vi "Initialize.vi"(7 "ProjectItem":refnum<class "ProjectItem.lvclass">, 8 "error in (no error)":errorcluster, 10 "New Name":string="NewName", 11 "Pattern":string="[Rename]") -> (0 "error out":errorcluster, 3 "ProjectItem out":refnum<class "ProjectItem.lvclass">)   [LabVIEW 2019, in "ProjectItem.lvclass"]
uses:
  ProjectItem.lvclass
  ProjectItem.lvclass/ProjectItem.ctl
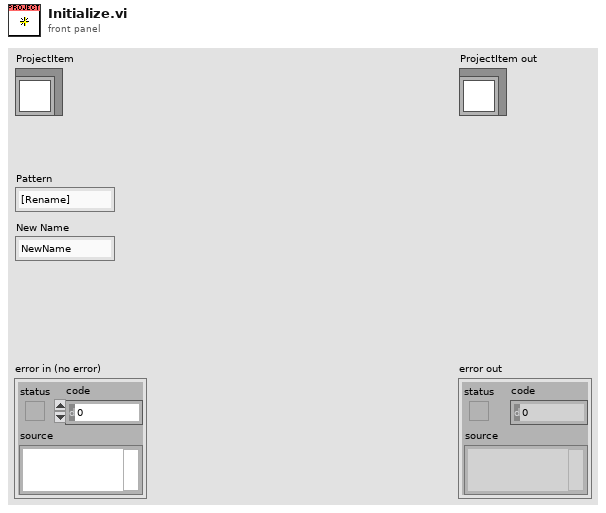
[diagram p1: front panel]
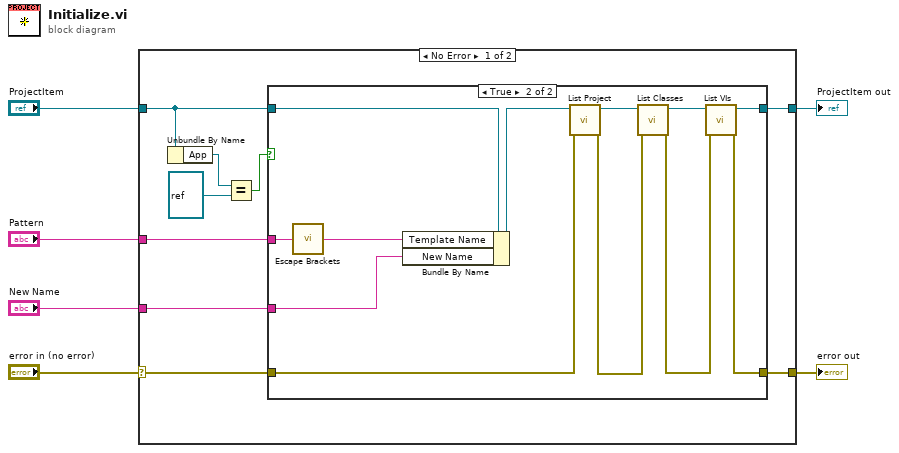
[diagram p0: block diagram]
diagram:
  n1 = case shown="No Error" "error in (no error)" {
    selector: "error in (no error)" -> [w15 w31]
    tunnel: [w13 w31] -> w5
    tunnel: [w14 w30] -> w3
    tunnel: "ProjectItem" -> [w10 w30]
    tunnel: "Pattern" -> [w12 _]
    tunnel: "New Name" -> [w11 _]
    frame No Error {
      n2 = Unbundle By Name(w10) -> ("App"=w9:refnum<vi>)
      n3 = Equal?(x=w9, y=refnum<vi> refnum ("App")) -> (x = y?=w8:bool)
      n4 = case shown="True" w8 {
        tunnel: w15 -> [w16 w21]
        tunnel: [w17 w26] -> w14
        tunnel: [w16 w24] -> w13
        tunnel: w12 -> [_ w29]
        tunnel: w11 -> [_ w18]
        tunnel: w10 -> [w17 w20]
        frame False {
        }
        frame True {
          n5 = call "Escape Brackets.vi"("Pattern"=w29) -> ("result string"=w22:string)
          n6 = Bundle By Name(cluster=w20, "Template Name"=w22, "New Name"=w18) -> (w19:refnum<class "ProjectItem.lvclass">)
          n7 = call "List Project.vi"("error in (no error)"=w21, "Rename in"=w19) -> ("error out"=w23:errorcluster, "Rename out"=w28:refnum<class "ProjectItem.lvclass">)  [unwired: 8 in]
          n8 = call "List Classes.vi"("error in (no error)"=w23, "Rename in"=w28) -> ("error out"=w25:errorcluster, "Rename out"=w27:refnum<class "ProjectItem.lvclass">)  [unwired: 8 in]
          n9 = call "List VIs.vi"("error in (no error)"=w25, "Rename in"=w27) -> ("error out"=w24:errorcluster, "Rename out"=w26:refnum<class "ProjectItem.lvclass">)  [unwired: 8 in]
        }
      }
    }
    frame Error {
    }
  }
  "error out" <- w5
  "ProjectItem out" <- w3
